vi "PCI1240U初始化.vi"() -> (0 "DevAxesCount":u32, 1 "旋转电机":u32, 2 "电动缸电机":u32, 3 "DeviceHandle":u32, 4 "调间隙电机":u32, 5 "进给电机":u32)   [LabVIEW 2013]
panel:
  out "Error Output":errorcluster
  out "Device Type 2":u16(ring) items=["PCI-1220 (M0)"]
  out "AxisOpened":bool
  in  "Device Type":u16(ring) items=["PCI-1240 (M0)"]
  out "DeviceNum List":u32[](array[numeric])
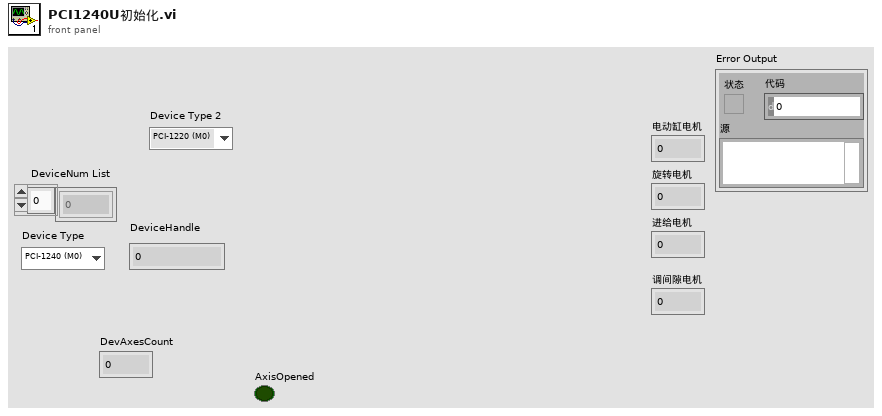
[diagram p1: front panel]
types:
  T1 = cluster{"DeviceNum":u32, "U*8 Array":cluster{"U*8 Array[0]":u8, "U*8 Array[1]":u8, "U*8 Array[2]":u8, "U*8 Array[3]":u8, "U*8 Array[4]":u8, "U*8 Array[5]":u8, "U*8 Array[6]":u8, "U*8 Array[7]":u8, "U*8 Array[8]":u8, "U*8 Array[9]":u8, "U*8 Array[10]":u8, "U*8 Array[11]":u8, "U*8 Array[12]":u8, "U*8 Array[13]":u8, "U*8 Array[14]":u8, "U*8 Array[15]":u8, "U*8 Array[16]":u8, "U*8 Array[17]":u8, "U*8 Array[18]":u8, "U*8 Array[19]":u8, "U*8 Array[20]":u8, "U*8 Array[21]":u8, "U*8 Array[22]":u8, "U*8 Array[23]":u8, "U*8 Array[24]":u8, "U*8 Array[25]":u8, "U*8 Array[26]":u8, "U*8 Array[27]":u8, "U*8 Array[28]":u8, "U*8 Array[29]":u8, "U*8 Array[30]":u8, "U*8 Array[31]":u8, "U*8 Array[32]":u8, "U*8 Array[33]":u8, "U*8 Array[34]":u8, "U*8 Array[35]":u8, "U*8 Array[36]":u8, "U*8 Array[37]":u8, "U*8 Array[38]":u8, "U*8 Array[39]":u8, "U*8 Array[40]":u8, "U*8 Array[41]":u8, "U*8 Array[42]":u8, "U*8 Array[43]":u8, "U*8 Array[44]":u8, "U*8 Array[45]":u8, "U*8 Array[46]":u8, "U*8 Array[47]":u8, "U*8 Array[48]":u8, "U*8 Array[49]":u8}, "NumOfSubDevice":i16}[]
  T2 = cluster{"U*8 Array[0]":u8, "U*8 Array[1]":u8, "U*8 Array[2]":u8, "U*8 Array[3]":u8, "U*8 Array[4]":u8, "U*8 Array[5]":u8, "U*8 Array[6]":u8, "U*8 Array[7]":u8, "U*8 Array[8]":u8, "U*8 Array[9]":u8, "U*8 Array[10]":u8, "U*8 Array[11]":u8, "U*8 Array[12]":u8, "U*8 Array[13]":u8, "U*8 Array[14]":u8, "U*8 Array[15]":u8, "U*8 Array[16]":u8, "U*8 Array[17]":u8, "U*8 Array[18]":u8, "U*8 Array[19]":u8, "U*8 Array[20]":u8, "U*8 Array[21]":u8, "U*8 Array[22]":u8, "U*8 Array[23]":u8, "U*8 Array[24]":u8, "U*8 Array[25]":u8, "U*8 Array[26]":u8, "U*8 Array[27]":u8, "U*8 Array[28]":u8, "U*8 Array[29]":u8, "U*8 Array[30]":u8, "U*8 Array[31]":u8, "U*8 Array[32]":u8, "U*8 Array[33]":u8, "U*8 Array[34]":u8, "U*8 Array[35]":u8, "U*8 Array[36]":u8, "U*8 Array[37]":u8, "U*8 Array[38]":u8, "U*8 Array[39]":u8, "U*8 Array[40]":u8, "U*8 Array[41]":u8, "U*8 Array[42]":u8, "U*8 Array[43]":u8, "U*8 Array[44]":u8, "U*8 Array[45]":u8, "U*8 Array[46]":u8, "U*8 Array[47]":u8, "U*8 Array[48]":u8, "U*8 Array[49]":u8}
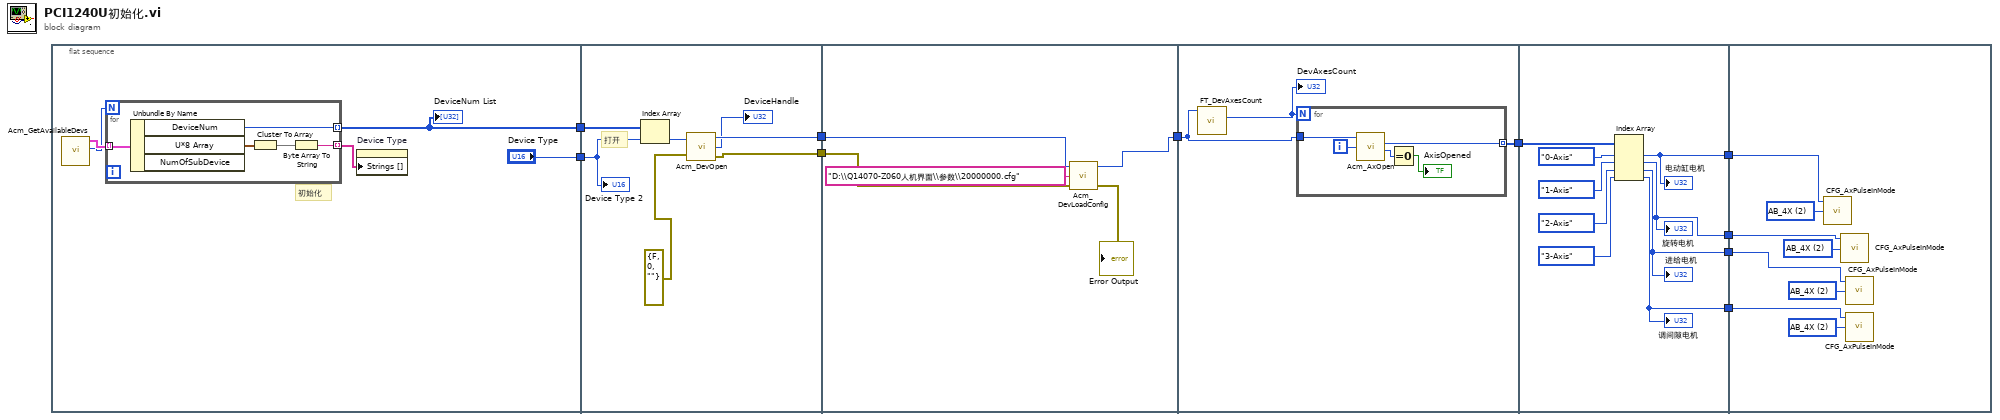
[diagram p0: block diagram]
diagram:
  n1 = flat-sequence {
    tunnel: [w14] -> w10
    tunnel: ["Device Type"] -> w9
    tunnel: w10 -> [w27]
    tunnel: w9 -> [w23]
    tunnel: [w25] -> w3
    tunnel: [w21] -> w1
    tunnel: w3 -> [w32]
    tunnel: [w30] -> w2
    tunnel: w1 -> [w29]
    tunnel: w2 -> [w34]
    tunnel: [w33] -> w8
    tunnel: w8 -> [w49]
    tunnel: [w47] -> w7
    tunnel: [w43] -> w6
    tunnel: [w42] -> w5
    tunnel: [w41] -> w4
    tunnel: w7 -> [w50]
    tunnel: w6 -> [w53]
    tunnel: w5 -> [w52]
    tunnel: w4 -> [w51]
    frame #0 {
      # "初始化"
      n2 = call <userlib>:"Acm_GetAvailableDevs.vi"() -> ("OutEntries"=w11:u32, "DeviceList"=w12:T1)  [unwired: 1 in, 2 out]
      n3 = for {
        N: w11 -> [_]
        tunnel: w12 -> [w20] mode=indexing
        tunnel: [w17] -> w14 mode=indexing
        tunnel: [w16] -> w15 mode=indexing
        n4 = Unbundle By Name(w20) -> ("DeviceNum"=w17:u32, "U*8 Array"=w19:T2)  [unwired: 1 out]
        n5 = Cluster To Array(cluster=w19) -> (array=w18:u8[])
        n6 = Byte Array To String(unsigned byte array=w18) -> (string=w16:string)
      }
      "DeviceNum List" <- w14
      n7 = property on="Device Type" class="Ring (严格)"("Strings []"=w15) -> ()  [unwired: 2 in, 2 out]
    }
    frame #1 {
      # "打开"
      n8 = Index Array(array=w27, index=w23) -> (element=w26:u32)
      n9 = call <userlib>:"Acm_DevOpen.vi"("Error Input(No Error)"=errorcluster {"status"=FALSE, "code"=0, "source"=""}, "DeviceNumber"=w26) -> ("Error Output"=w21:errorcluster, "ReturnValue"=→"DeviceHandle":u32, "DeviceHandle"=w25:u32)
      "Device Type 2" <- w23
    }
    frame #2 {
      n10 = call <userlib>:"Acm_DevLoadConfig.vi"("Error Input(No Error)"=w29, "ConfigPath"="D:\\Q14070-Z060人机界面\\参数\\20000000.cfg", "DeviceHandle"=w32) -> ("Error Output"=→"Error Output":errorcluster, "DeviceHandle"=w30:u32)  [unwired: 1 out]
    }
    frame #3 {
      n11 = call <userlib>:"FT_DevAxesCount.vi"("Handle"=w34) -> ("DevAxesCount"=w35:u32)  [unwired: 3 in, 4 out]
      "DevAxesCount" <- w35
      n12 = for {
        N: w35 -> [_]
        tunnel: w34 -> [w40]
        tunnel: [w36] -> w33 mode=indexing
        i -> [w39]
        n13 = call <userlib>:"Acm_AxOpen.vi"("PhyAxis"=w39, "DeviceHandle"=w40) -> ("ReturnValue"=w38:u32, "AxisHandle"=w36:u32)  [unwired: 1 in, 2 out]
        n14 = Equal To 0?(x=w38) -> (x = 0?=→"AxisOpened":bool)
      }
    }
    frame #4 {
      n15 = Index Array(array=w49, index #1=enum32{"0-Axis", "1-Axis", "2-Axis", "3-Axis"}."0-Axis" ("Operate Axis"), index #2=enum32{"0-Axis", "1-Axis", "2-Axis", "3-Axis"}."1-Axis" ("Operate Axis"), index #3=enum32{"0-Axis", "1-Axis", "2-Axis", "3-Axis"}."2-Axis" ("Operate Axis"), index #4=enum32{"0-Axis", "1-Axis", "2-Axis", "3-Axis"}."3-Axis" ("Operate Axis")) -> (element #1=w47:u32, element #2=w43:u32, element #3=w42:u32, element #4=w41:u32)
      "电动缸电机" <- w47
      "旋转电机" <- w43
      "进给电机" <- w42
      "调间隙电机" <- w41
    }
    frame #5 {
      w54 = u32 2 items=["AB_1X", "AB_2X", "AB_4X", "I_CW_CCW"] ("CFG_AxPulseInMode")
      w55 = u32 2 items=["AB_1X", "AB_2X", "AB_4X", "I_CW_CCW"] ("CFG_AxPulseInMode")
      w56 = u32 2 items=["AB_1X", "AB_2X", "AB_4X", "I_CW_CCW"] ("CFG_AxPulseInMode")
      w57 = u32 2 items=["AB_1X", "AB_2X", "AB_4X", "I_CW_CCW"] ("CFG_AxPulseInMode")
      n16 = call <userlib>:"CFG_AxPulseInMode.vi"("CFG_AxPulseInMode"=w57, "Handle"=w50) -> ()  [unwired: 1 in, 3 out]
      n17 = call <userlib>:"CFG_AxPulseInMode.vi"("CFG_AxPulseInMode"=w56, "Handle"=w53) -> ()  [unwired: 1 in, 3 out]
      n18 = call <userlib>:"CFG_AxPulseInMode.vi"("CFG_AxPulseInMode"=w55, "Handle"=w52) -> ()  [unwired: 1 in, 3 out]
      n19 = call <userlib>:"CFG_AxPulseInMode.vi"("CFG_AxPulseInMode"=w54, "Handle"=w51) -> ()  [unwired: 1 in, 3 out]
    }
  }
